vi "write_checkpoint_specfile.vi"() -> ()   [LabVIEW 2019]
uses:
  lib/libSimulationControl/libSimulationControl.lvlib
panel:
  out "Old Specification":path
  out "Working Directory":path
  out "New Specification":path
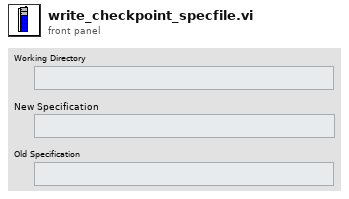
[diagram p1: front panel]
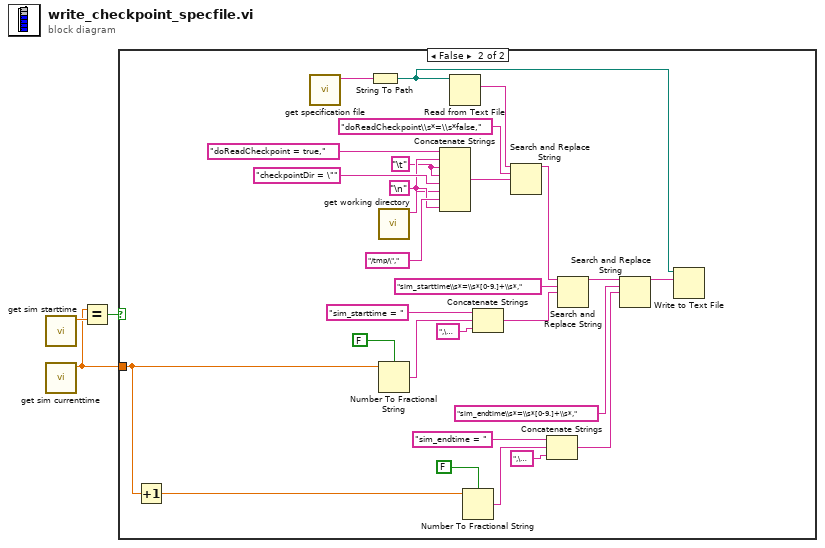
[diagram p0: block diagram]
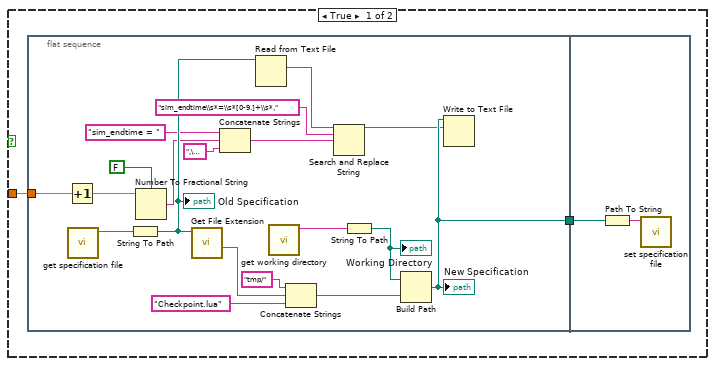
[diagram p2: hidden frame]
diagram:
  n1 = call "get sim starttime.vi"() -> ("function return"=w2:dbl)  [unwired: 10 in, 1 out]
  n2 = call "get sim currenttime.vi"() -> ("function return"=w1:dbl)  [unwired: 10 in, 1 out]
  n3 = Equal?(x=w1, y=w2) -> (x = y?=w3:bool)
  n4 = case shown="False" w3 {
    tunnel: w1 -> [w4 w54]
    frame True {
      n5 = flat-sequence {
        tunnel: [w20] -> w5
        tunnel: w4 -> [w18]
        tunnel: w5 -> [w26]
        frame #0 {
          n6 = Increment(x=w18) -> (x+1=w11:dbl)
          n7 = call "get specification file.vi"() -> ("function return"=w7:string)  [unwired: 10 in, 1 out]
          n8 = String To Path(string=w7) -> (path=w21:path)
          "Old Specification" <- w21
          n9 = Number To Fractional String(use system decimal point (T)=FALSE, number=w11) -> (F-format string=w16:string)  [unwired: 2 in]
          n10 = call <vilib>:"Get File Extension.vi"("file"=w21) -> ("filename without extension"=w22:string)  [unwired: 6 in, 4 out]
          n11 = Concatenate Strings("sim_endtime = " ("replace string (\"\")"), w16, ",\u0000\\n" ("string")) -> (w14:string)
          n12 = Read from Text File(file (use dialog)=w21) -> (text=w10:string)  [unwired: 3 in, 3 out]
          n13 = call "get working directory.vi"() -> ("function return"=w6:string)  [unwired: 10 in, 1 out]
          n14 = Concatenate Strings("tmp/" ("string"), w22, "Checkpoint.lua" ("string")) -> (w23:string)
          n15 = Search and Replace String(input string=w10, search string="sim_endtime\\s*=\\s*[0-9.]+\\s*,", replace string=w14) -> (result string=w13:string)  [unwired: 5 in, 3 out]
          n16 = String To Path(string=w6) -> (path=w8:path)
          "Working Directory" <- w8
          n17 = Build Path(base path=w8, name or relative path=w23) -> (appended path=w20:path)
          "New Specification" <- w20
          n18 = Write to Text File(file (use dialog)=w20, text=w13) -> ()  [unwired: 2 in, 3 out]
        }
        frame #1 {
          n19 = Path To String(path=w26) -> (string=w25:string)
          n20 = call "set specification file.vi"("spec_file"=w25) -> ()  [unwired: 10 in, 1 out]
        }
      }
    }
    frame False {
      w46 = "\t"
      w47 = "\n"
      n21 = Increment(x=w54) -> (x+1=w53:dbl)
      n22 = call "get specification file.vi"() -> ("function return"=w28:string)  [unwired: 10 in, 1 out]
      n23 = String To Path(string=w28) -> (path=w29:path)
      n24 = call "get working directory.vi"() -> ("function return"=w27:string)  [unwired: 10 in, 1 out]
      n25 = Number To Fractional String(use system decimal point (T)=FALSE, number=w54) -> (F-format string=w42:string)  [unwired: 2 in]
      n26 = Concatenate Strings("doReadCheckpoint = true," ("search string"), w47, w46, w46, "checkpointDir = \"" ("string"), w27, "/tmp/\"," ("string"), w47) -> (w50:string)
      n27 = Read from Text File(file (use dialog)=w29) -> (text=w30:string)  [unwired: 3 in, 3 out]
      n28 = Number To Fractional String(use system decimal point (T)=FALSE, number=w53) -> (F-format string=w37:string)  [unwired: 2 in]
      n29 = Concatenate Strings("sim_starttime = " ("replace string (\"\")"), w42, ",\u0000\\n" ("string")) -> (w44:string)
      n30 = Search and Replace String(input string=w30, search string="doReadCheckpoint\\s*=\\s*false,", replace string=w50) -> (result string=w40:string)  [unwired: 5 in, 3 out]
      n31 = Concatenate Strings("sim_endtime = " ("replace string (\"\")"), w37, ",\u0000\\n" ("string")) -> (w35:string)
      n32 = Search and Replace String(input string=w40, search string="sim_starttime\\s*=\\s*[0-9.]+\\s*,", replace string=w44) -> (result string=w34:string)  [unwired: 5 in, 3 out]
      n33 = Search and Replace String(input string=w34, search string="sim_endtime\\s*=\\s*[0-9.]+\\s*,", replace string=w35) -> (result string=w33:string)  [unwired: 5 in, 3 out]
      n34 = Write to Text File(file (use dialog)=w29, text=w33) -> ()  [unwired: 2 in, 3 out]
    }
  }
